vi "AddNode.vi"(8 "error in":errorcluster, 9 "parameters":variant, 10 "parent node ID":string, 11 "CEF_Node in":refnum<class "CEF_Node.lvclass">) -> (0 "error out":errorcluster, 2 "summary":T1[](array[typedef]))   [LabVIEW 2025, in "CEF.lvlib"]
doc: "This Vi adds a new node to the Parent Node IDCopyright 2017 National Instruments Corporation\n\nLicensed under the Apache License, Version 2.0 (the \"License\"); you may not use this file except in compliance with the License. You may obtain a copy of the License at http://www.apache.org/licenses/LICENSE-2.0\nUnless required by applicable law or agreed to in writing, software distributed under the License is distributed on an \"AS IS\" BASIS, WITHOUT WARRANTIES OR CONDITIONS OF ANY KIND, either express or implied. See the License for the specific language governing permissions and limitations under the License."
uses:
  CEF.lvlib
  Node/Summary.ctl
  Node/CEF_Node.lvclass
  Node/CEF_Node.lvclass/CEF_Node.ctl
  Node/ReadChildren.vi
  Node/WriteParent.vi
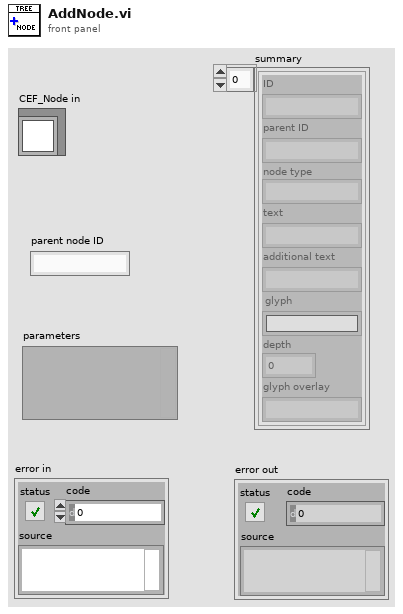
[diagram p1: front panel]
types:
  T1 = typedef "CEF.lvlib/CEF_Node.lvclass/Summary.ctl" = cluster{"ID":string, "parent ID":string, "node type":string, "text":string, "additional text":string, "glyph":string, "depth":i32, "glyph overlay":string}
  T2 = typedef "CEF.lvlib/CEF_Node.lvclass/NodeRef.ctl" = refnum<data-value>
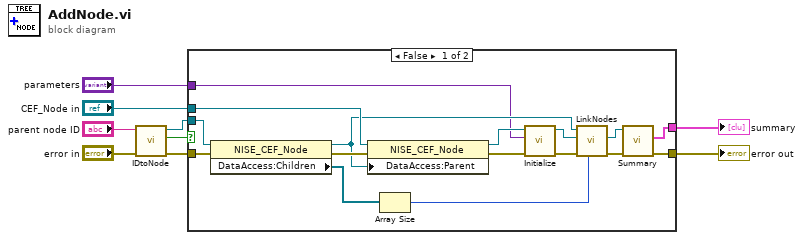
[diagram p0: block diagram]
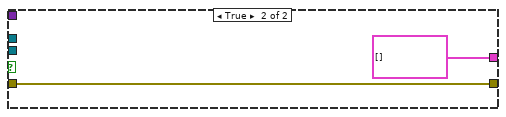
[diagram p2: hidden frame]
diagram:
  n1 = call "IDtoNode.vi"("error in"="error in", "ID"="parent node ID") -> ("error out"=w2:errorcluster, "invalid Id"=w1:bool, "node ref"=w3:T2)  [unwired: 7 in]
  n2 = case shown="False" w1 {
    tunnel: w3 -> [w19 _]
    tunnel: [w25 T1[] [] ("summary")] -> w7
    tunnel: [w24 w27] -> w6
    tunnel: "CEF_Node in" -> [w14 _]
    tunnel: w2 -> [w17 w27]
    tunnel: "parameters" -> [w10 _]
    frame False {
      n3 = property class="NISE_CEF_Node"(reference=w19, error in=w17) -> (reference out=w12:T2, error out=w16:errorcluster, "DataAccess:Children"=w18:T2[])
      n4 = property class="NISE_CEF_Node"(reference=w14, error in=w16, "DataAccess:Parent"=w12) -> (reference out=w13:refnum<class "CEF_Node.lvclass">, error out=w15:errorcluster)
      n5 = Array Size(array=w18) -> (size(s)=w11:i32)
      n6 = call-dynamic "Initialize.vi"("error in"=w15, "parameters"=w10, "CEF_Node in"=w13) -> ("error out"=w20:errorcluster, "data value reference"=w21:T2)  [unwired: 6 in, 1 out]
      n7 = call "LinkNodes.vi"("index"=w11, "error in"=w20, "child in"=w21, "parent in"=w12) -> ("error out"=w23:errorcluster, "child out"=w22:T2)  [unwired: 5 in, 1 out]
      n8 = call "Summary.vi"("error in"=w23, "node self ref"=w22) -> ("error out"=w24:errorcluster, "summary"=w25:T1[])  [unwired: 8 in]
    }
    frame True {
    }
  }
  "error out" <- w6
  "summary" <- w7
